vi "CreateSystemReference.vi"() -> (0 "error out":errorcluster, 3 "Cluster":T1)   [LabVIEW 2013]
uses:
  Control/SystemData.ctl
  Control/SignalType.ctl
  Control/SystemCommand.ctl
  Control/SubDaqCommand.ctl
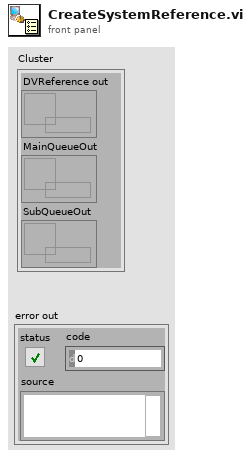
[diagram p1: front panel]
types:
  T1 = cluster{"DVReference out":refnum<data-value>, "MainQueueOut":refnum<queue>, "SubQueueOut":refnum<queue>}
  T2 = typedef "SubDaqCommand.ctl" = enum16{"None", "Init", "Work", "Stop", "Close"}
  T3 = typedef "SystemCommand.ctl" = enum16{"None", "Init", "Close", "ShowNumeric", "ShowString", "ShowBool", "SquareNumeric", "ReverseString", "InvertBool", "FFT"}
  T4 = typedef "SystemData.ctl" = cluster{"Numeric":dbl, "String":string, "Boolean":bool, "Frequency":dbl, "Amplitude":dbl, "SignalType":T5, "WaveformArray":waveform(dbl)[], "Reset":bool, "StateString":string, "FFTmagnitudes":cluster{"f0":dbl, "df":dbl, "magnitude":dbl[]}[]}
  T5 = typedef "SignalType.ctl" = enum16{"Sin", "Triangle", "Square"}
  T6 = cluster{"data value reference":refnum<data-value>, "queue out":refnum<queue>, "queue out":refnum<queue>}
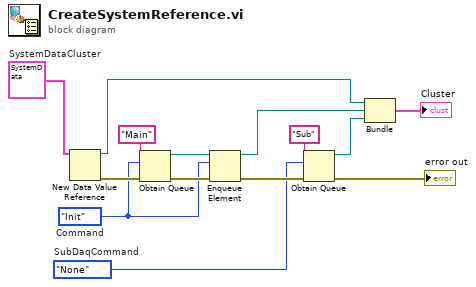
[diagram p0: block diagram]
diagram:
  w6 = SubDaqCommand."None"  # SubDaqCommand
  w10 = SystemCommand."Init"  # Command
  w14 = T4 {"Numeric"=0.0, "String"="", "Boolean"=FALSE, "Frequency"=0.0, "Amplitude"=0.0, "SignalType"=enum."Sin", "WaveformArray"=[], "Reset"=FALSE, "StateString"="", "FFTmagnitudes"=[]}  # SystemDataCluster
  n1 = New Data Value Reference(data value=w14) -> (data value reference=w3:refnum<data-value>, error out=w13:errorcluster)  [unwired: 1 in]
  n2 = Obtain Queue(name (unnamed)="Main", element data type=w10, error in (no error)=w13) -> (queue out=w12:refnum<queue>, error out=w11:errorcluster)  [unwired: 2 in, 1 out]
  n3 = Enqueue Element(queue=w12, element=w10, error in (no error)=w11) -> (queue out=w4:refnum<queue>, error out=w7:errorcluster)  [unwired: 1 in, 1 out]
  n4 = Obtain Queue(name (unnamed)="Sub", element data type=w6, error in (no error)=w7) -> (queue out=w2:refnum<queue>, error out=→"error out":errorcluster)  [unwired: 2 in, 1 out]
  n5 = Bundle("data value reference"=w3, "queue out"=w4, "queue out"=w2) -> (→"Cluster":T6)  [unwired: 1 in]
